vi "Cannon manual control.vi"() -> ()   [LabVIEW 2012]
panel:
  out "Current angle 2":dbl
  out "Motor value":dbl
  out "On target":bool
  in  "Throttle value":dbl
  in  "Current angle":dbl
  in  "Min Angle":dbl
  in  "Max Angle":dbl
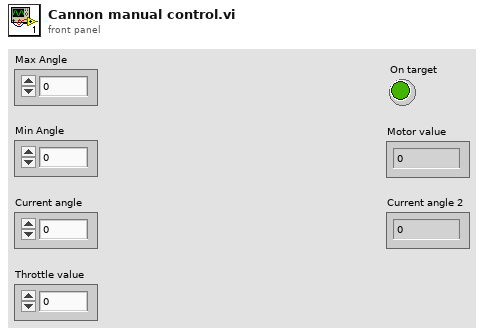
[diagram p1: front panel]
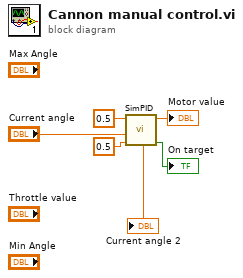
[diagram p0: block diagram]
diagram:
  n1 = call "SimPID.vi"("Range"=0.5, "Position"="Current angle", "Gain"=0.5) -> ("On Target"=→"On target":bool, "result"=→"Motor value":dbl)  [unwired: 6 in]
  "Current angle 2" <- "Current angle"
